vi "niFPGA Shift 3 Saturate (to I16).vi"(2 "I32 input":i32 format="%08x") -> (6 "saturated I16 output":i16 format="%.0x")   [LabVIEW 2017]
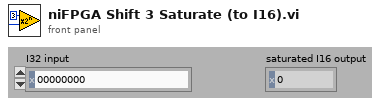
[diagram p1: front panel]
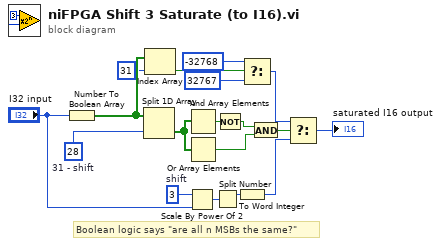
[diagram p0: block diagram]
diagram:
  w18 = i8 3  # shift
  w17 = i8 28  # 31 - shift
  # "Boolean logic says \"are all n MSBs the same?\""
  n1 = Number To Boolean Array(number="I32 input") -> (Boolean array=w13:bool[])
  n2 = Split 1D Array(array=w13, index=w17) -> (second subarray=w14:bool[])  [unwired: 1 out]
  n3 = Index Array(array=w13, index=31) -> (element=w11:bool)
  n4 = Scale By Power Of 2(n=w18, x="I32 input") -> (x*2^n=w15:i32)
  n5 = And Array Elements(Boolean array=w14) -> (logical AND=w6:bool)
  n6 = Or Array Elements(Boolean array=w14) -> (logical OR=w4:bool)
  n7 = Split Number(x=w15) -> (hi(x)=w10:u16)  [unwired: 1 out]
  n8 = Not(x=w6) -> (.not. x?=w5:bool)
  n9 = To Word Integer(number=w10) -> (16bit integer=w1:i16)
  n10 = Select(t=i16 -32768, s=w11, f=i16 32767) -> (s? t:f=w2:i16)
  n11 = And(x=w5, y=w4) -> (x .and. y?=w3:bool)
  n12 = Select(t=w2, s=w3, f=w1) -> (s? t:f=→"saturated I16 output":i16)
